vi "ValidateFileConfigDTO.vi"(8 "error in (no error)":errorcluster, 11 "FileConfigDTOin":T1) -> (0 "error out":errorcluster, 3 "FileConfigDTOout":T1)   [LabVIEW 2026, in "Lumberjack.lvlib"]
uses:
  Lumberjack.lvlib
  TypeDefs/ConfigDTO/FileConfigDTO.ctl
  <vilib>/Utility/Data Type/NI_Data Type.lvlib
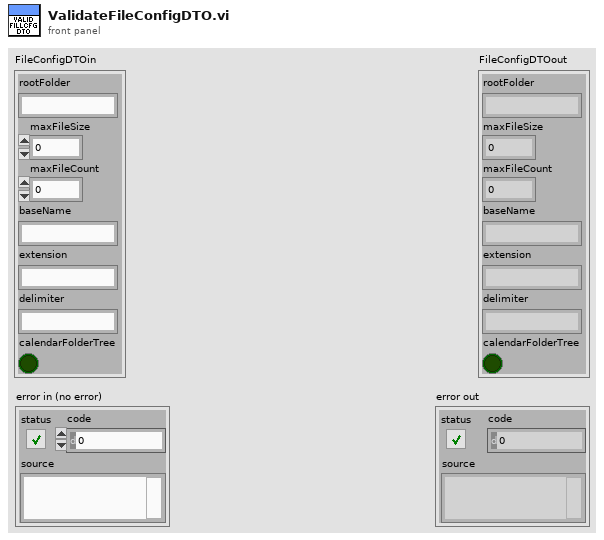
[diagram p1: front panel]
types:
  T1 = typedef "Lumberjack.lvlib/FileConfigDTO.ctl" = cluster{"rootFolder":string, "maxFileSize":i64, "maxFileCount":i32, "baseName":string, "extension":string, "delimiter":string, "calendarFolderTree":bool}
  T2 = typedef "NI_Data Type.lvlib/Data Type.ctl" = enum8{"Invalid Type", "Void", "I8", "I16", "I32", "I64", "U8", "U16", "U32", "U64", "Single Float", "Double Float", "Extended Float", "Single Complex", "Double Complex", "Extended Complex", "Enum U8", "Enum U16", "Enum U32", "Enum U64", "Single Float With Unit", "Double Float With Unit", "Extended Float With Unit", "Single Complex with Unit", "Double Complex with Unit", "Extended Complex with Unit", "Boolean", "String", "Path", "Picture", "Tag", "Array", "Cluster", "Variant", "LV Variant", "Waveform", "Timestamp", "Digital Waveform", "Digital Data", "ExpressData", "Refnum", "External Data", "VI", "Poly VI", "LabVIEW Class Instance", "Fixed Point", "Set Collection", "Map Collection"}
  T3 = typedef "NI_Data Type.lvlib/Type Definition Info.ctl" = cluster{"Name":string, "Timestamp":u32}
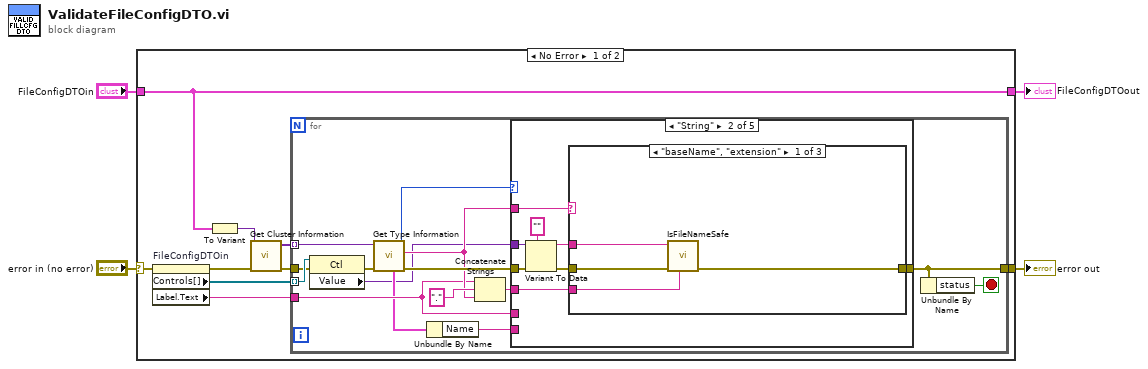
[diagram p0: block diagram]
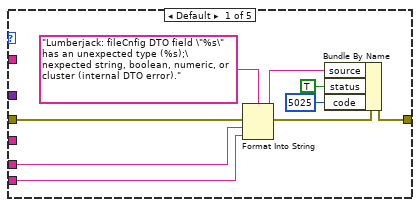
[diagram p2: hidden frame]
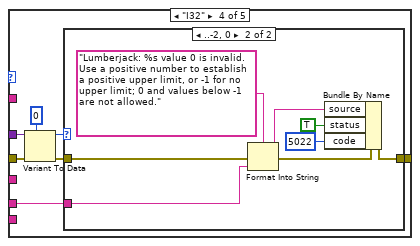
[diagram p6: hidden frame]
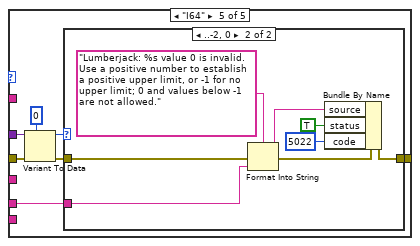
[diagram p8: hidden frame]
diagram:
  n1 = case shown="No Error" "error in (no error)" {
    selector: "error in (no error)" -> [w8 w85]
    tunnel: [w10 w85] -> w4
    tunnel: "FileConfigDTOin" -> [w9 w86]
    tunnel: [w9 w86] -> w2
    frame No Error {
      n2 = property on="FileConfigDTOin" class="Clust (strict)"(error in=w8) -> (error out=w7:errorcluster, "Controls[]"=w6:refnum<vi>[], "Label.Text"=w5:string)  [unwired: 1 in, 1 out]
      n3 = To Variant(anything=w9) -> (Variant=w11:variant)
      n4 = call <vilib>:"Get Cluster Information.vi"("error in (no error)"=w7, "variant"=w11) -> ("error out"=w12:errorcluster, "cluster elements"=w13:variant[])  [unwired: 8 in]
      n5 = for {
        tunnel: w13 -> [w23] mode=indexing
        tunnel: w12 -> [w16]
        tunnel: w5 -> [w22]
        tunnel: [w19] -> w10
        tunnel: w6 -> [w17] mode=indexing
        stop <- w18 stop-if-true
        n6 = property class="Ctl"(reference=w17, error in=w16) -> (error out=w14:errorcluster, "Value"=w15:variant)  [unwired: 1 out]
        n7 = call <vilib>:"Get Type Information.vi"("error in (no error)"=w14, "variant"=w23) -> ("error out"=w27:errorcluster, "name"=w24:string, "type"=w25:T2, "type definition info"=w21:T3)  [unwired: 5 in, 1 out]
        n8 = Unbundle By Name(w21) -> ("Name"=w20:string)
        n9 = Concatenate Strings(w22, "." ("string"), w24) -> (w26:string)
        n10 = case shown="\"String\"" w25 {
          tunnel: w27 -> [w33 w43 w52 w57 w73]
          tunnel: w26 -> [_ w45 _ _ _]
          tunnel: w24 -> [_ w44 _ _ _]
          tunnel: w15 -> [_ w41 _ w55 w71]
          tunnel: w22 -> [w34 _ _ w58 w74]
          tunnel: [w30 w38 w52 w59 w75] -> w19
          tunnel: w20 -> [w31 _ _ _ _]
          frame Default {
            n11 = Format Into String(format string="Lumberjack: fileCnfig DTO field \"%s\" has an unexpected type (%s);\nexpected string, boolean, numeric, or cluster (internal DTO error)." ("source"), error in=w33, w34, w31) -> (resulting string=w29:string, error out=w32:errorcluster)  [unwired: 1 in]
            n12 = Bundle By Name(cluster=w32, "source"=w29, "status"=TRUE, "code"=5025) -> (w30:errorcluster)
          }
          frame "String" {
            n13 = Variant To Data(error in=w43, type="", Variant=w41) -> (data=w39:string, error out=w42:errorcluster)
            n14 = case shown="\"baseName\", \"extension\"" w44 {
              tunnel: w42 -> [w49 w50 w51]
              tunnel: w45 -> [w48 _ _]
              tunnel: w39 -> [w47 _ _]
              tunnel: [w46 w50 w51] -> w38
              frame "baseName", "extension" {
                n15 = call "IsFileNameSafe.vi"("Context"=w48, "error in (no error)"=w49, "candidate"=w47) -> ("error out"=w46:errorcluster)  [unwired: 6 in, 2 out]
              }
              frame "delimiter", "rootFolder" {
              }
              frame Default {
              }
            }
          }
          frame "Boolean" {
          }
          frame "I32" {
            n16 = Variant To Data(error in=w57, type=0, Variant=w55) -> (data=w53:i32, error out=w56:errorcluster)
            n17 = case shown="..-2, 0" w53 {
              tunnel: [w60 w66] -> w59
              tunnel: w56 -> [w60 w65]
              tunnel: w58 -> [_ w61]
              frame Default {
              }
              frame ..-2, 0 {
                n18 = Format Into String(format string="Lumberjack: %s value 0 is invalid. Use a positive number to establish a positive upper limit, or -1 for no upper limit; 0 and values below -1 are not allowed." ("source"), error in=w65, w61) -> (resulting string=w63:string, error out=w64:errorcluster)  [unwired: 1 in]
                n19 = Bundle By Name(cluster=w64, "source"=w63, "status"=TRUE, "code"=5022) -> (w66:errorcluster)
              }
            }
          }
          frame "I64" {
            n20 = Variant To Data(error in=w73, type=i64 0, Variant=w71) -> (data=w69:i64, error out=w72:errorcluster)
            n21 = case shown="..-2, 0" w69 {
              tunnel: [w76 w82] -> w75
              tunnel: w72 -> [w76 w81]
              tunnel: w74 -> [_ w77]
              frame Default {
              }
              frame ..-2, 0 {
                n22 = Format Into String(format string="Lumberjack: %s value 0 is invalid. Use a positive number to establish a positive upper limit, or -1 for no upper limit; 0 and values below -1 are not allowed." ("source"), error in=w81, w77) -> (resulting string=w79:string, error out=w80:errorcluster)  [unwired: 1 in]
                n23 = Bundle By Name(cluster=w80, "source"=w79, "status"=TRUE, "code"=5022) -> (w82:errorcluster)
              }
            }
          }
        }
        n24 = Unbundle By Name(w19) -> ("status"=w18:bool)
      }
    }
    frame Error {
    }
  }
  "error out" <- w4
  "FileConfigDTOout" <- w2
